vi "Get Changed VIs.vi"(8 "error in":errorcluster, 10 "VIs":string[](array[string]), 11 "Application in":refnum<vi>) -> (0 "error out":errorcluster, 1 "Changed Items":T1(array[cluster]), 2 "Items no longer in memory":string[](array[string]), 4 "Canceled":bool)   [LabVIEW 2013, in "LVTM.lvlib"]
uses:
  LVTM.lvlib
panel:
  out "Unsasved VIs":string[](array[string])
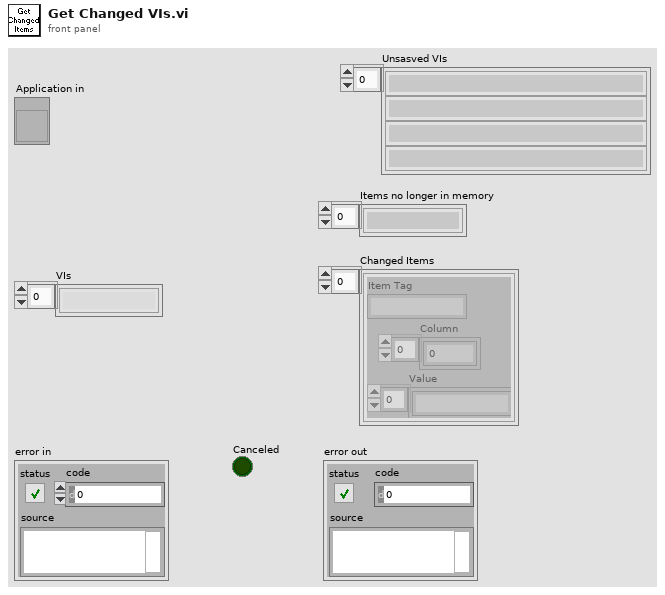
[diagram p1: front panel]
types:
  T1 = cluster{"Item Tag":string, "Column":i32[], "Value":string[]}[]
  T2 = cluster{"Item Tag":string, "Column":i32[], "Value":string[]}
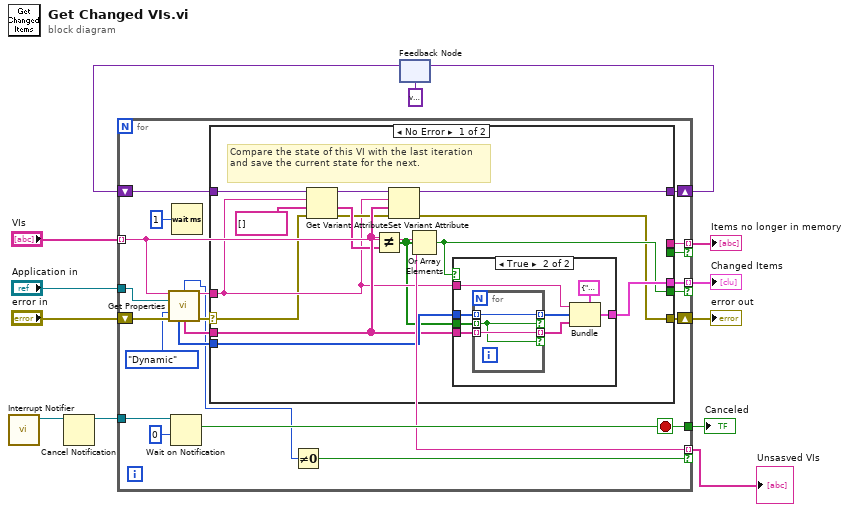
[diagram p0: block diagram]
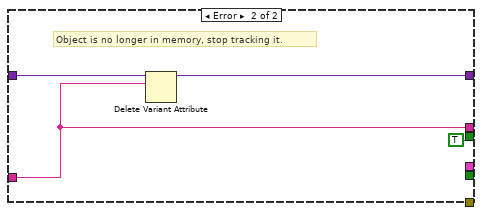
[diagram p3: hidden frame]
diagram:
  n1 = call "Interrupt Notifier.vi"() -> ("Notifier out"=w4:refnum<notifier>)  [unwired: 10 in, 1 out]
  n2 = Cancel Notification(0:w4) -> (8:w2:refnum<notifier>)  [unwired: 1 in, 2 out]
  n3 = feedback #1(variant ("Variant")) -> (w6:variant)
  n4 = for {
    tunnel: "VIs" -> [w15] mode=indexing
    tunnel: "Application in" -> [w31]
    shift-right: [w26] -> w7
    shift-left: w6 -> [w27]
    tunnel: [w25] -> w11 mode=indexing if=w24
    tunnel: [w23] -> w10 mode=indexing if=w22
    shift-right: [w32] -> w9
    shift-left: "error in" -> [w34]
    tunnel: w2 -> [w18]
    tunnel: [w17] -> w3
    tunnel: [w15] -> w1 mode=indexing if=w14
    stop <- w17 stop-if-true
    n5 = call "Get Properties.vi"("VI Name"=w15, "AppInst"=w31, "Scope (0:All)"=enum16{"All", "Dynamic"}."Dynamic" ("Properties"), "error in"=w34) -> ("Modifications:VI Modifications Bitset"=w16:u64, "Full Name Out"=w33:string, "ColumnOffsets (Dyn)"=w28:i32[], "VI Properties (Dyn)"=w29:string[], "error out"=w30:errorcluster)  [unwired: 2 in, 5 out]
    n6 = Wait on Notification(notifier=w18, timeout in ms (-1)=0) -> (notification=w17:bool)  [unwired: 2 in, 3 out]
    n7 = Wait (ms)(milliseconds to wait=u32 1) -> ()  [unwired: 1 out]
    n8 = case shown="No Error" w30 {
      selector: w30 -> [w36 _]
      tunnel: w33 -> [w40 w61]
      tunnel: w29 -> [w43 _]
      tunnel: [w35 _] -> w32
      tunnel: w28 -> [w48 _]
      tunnel: w27 -> [w46 w63]
      tunnel: [w47 w62] -> w26
      tunnel: [w39 _] -> w25
      tunnel: [w37 _] -> w24
      tunnel: [_ w61] -> w23
      tunnel: [_ TRUE] -> w22
      frame No Error {
        # "Compare the state of this VI with the last iteration and save the current state for the next."
        n9 = Get Variant Attribute(Variant=w46, name=w40, default value (empty Variant)=string[] [] ("VI Properties (Dyn)"), error in=w36) -> (duplicate Variant=w44:variant, value=w42:string[], error out=w41:errorcluster)  [unwired: 1 out]
        n10 = Not Equal?(x=w43, y=w42) -> (x != y?=w38:bool[])
        n11 = Set Variant Attribute(Variant=w44, name=w40, value=w43, error in=w41) -> (Variant out=w47:variant, error out=w35:errorcluster)  [unwired: 1 out]
        n12 = Or Array Elements(Boolean array=w38) -> (logical OR=w37:bool)
        n13 = case shown="True" w37 {
          tunnel: w48 -> [_ w56]
          tunnel: w43 -> [_ w55]
          tunnel: w40 -> [_ w52]
          tunnel: [_ w50] -> w39
          tunnel: w38 -> [_ w49]
          frame False {
          }
          frame True {
            n14 = for {
              tunnel: w55 -> [w58] mode=indexing
              tunnel: w56 -> [w59] mode=indexing
              tunnel: w49 -> [w57] mode=indexing
              tunnel: [w59] -> w54 mode=indexing if=w57
              tunnel: [w58] -> w53 mode=indexing if=w57
            }
            n15 = Bundle(cluster=T2 {"Item Tag"="", "Column"=[], "Value"=[]}, "Item Tag"=w52, "Column"=w54, "Value"=w53) -> (w50:T2)
          }
        }
      }
      frame Error {
        # "Object is no longer in memory, stop tracking it."
        n16 = Delete Variant Attribute(6:w61, 7:w63) -> (3:w62:variant)  [unwired: 1 in, 2 out]
      }
    }
    n17 = Not Equal To 0?(x=w16) -> (x != 0?=w14:bool)
  }
  "Changed Items" <- w11
  "Items no longer in memory" <- w10
  "error out" <- w9
  "Canceled" <- w3
  "Unsasved VIs" <- w1
  n18 = feedback-in #1(w7) -> ()
